vi "LaserLineDetection_Intensity_Gauss.vi"(6 "Color":u32(colorbox)=16744448, 8 "Error In":errorcluster, 10 "Point Information In":T1, 11 "Source In":T2=refnum) -> (0 "Error Out":errorcluster, 1 "appended array":cluster{u8[], i32[]}[](array[cluster]), 2 "Point Information Out":T1, 3 "Source Out":T2, 4 "Gauss Fit Accepted":bool, 5 "Intensity Average":u8)   [LabVIEW 2013]
uses:
  <vilib>/vision/Image Controls.llb/IMAQ Image.ctl
  Point Information.ctl
  <vilib>/Analysis/6fits.llb/Curve Fitting Criteria.ctl
  <vilib>/vision/NI_Vision_Development_Module.lvlib
  <vilib>/Analysis/NI_AALPro.lvlib
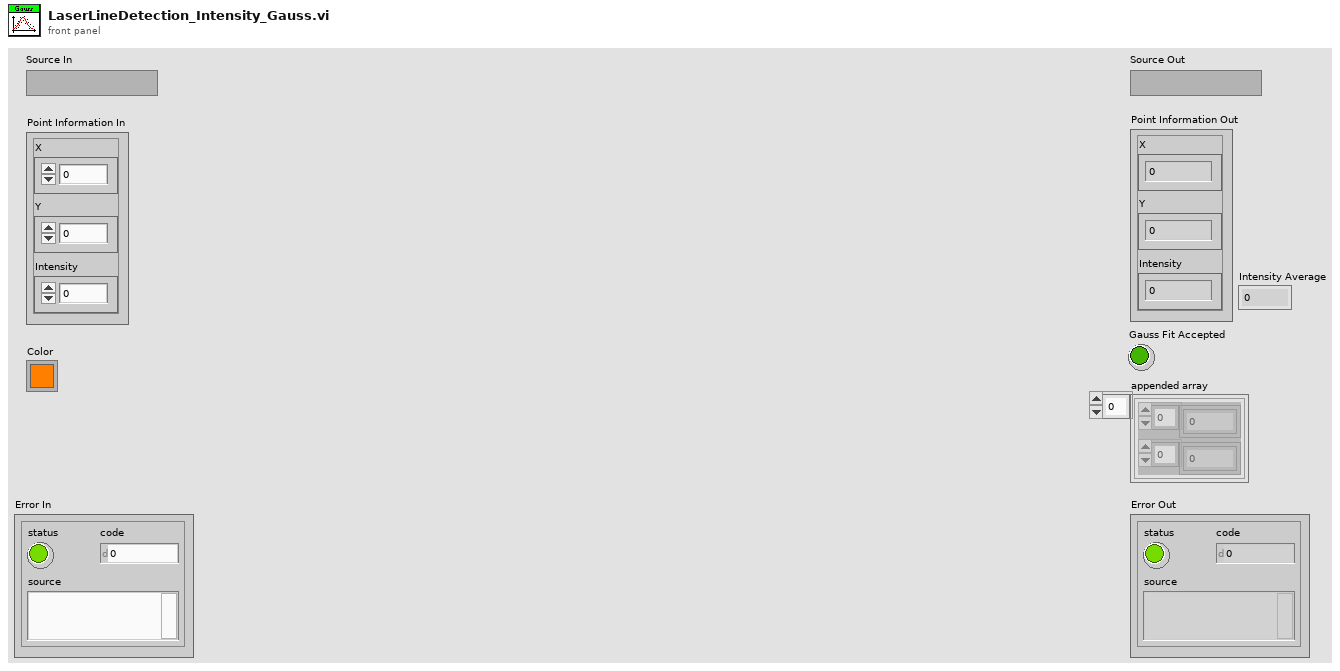
[diagram p1: front panel]
types:
  T1 = typedef "Point Information.ctl" = cluster{"X":i32, "Y":i32, "Intensity":u8}
  T2 = typedef "IMAQ Image.ctl" = refnum<image>
  T3 = cluster{"amp min":dbl, "amp max":dbl, "center min":dbl, "center max":dbl, "deviation min":dbl, "deviation max":dbl, "offset min":dbl, "offset max":dbl}
  T4 = typedef "NI_AALPro.lvlib/Curve Fitting Criteria.ctl" = u16
  T5 = cluster{"initial amplitude":dbl, "initial center":dbl, "initial standard deviation":dbl, "offset":dbl}
  T6 = cluster{"Red (or Hue) value":u8, "Green (or Sat) value":u8, "Blue (or Light or Val) value":u8}[]
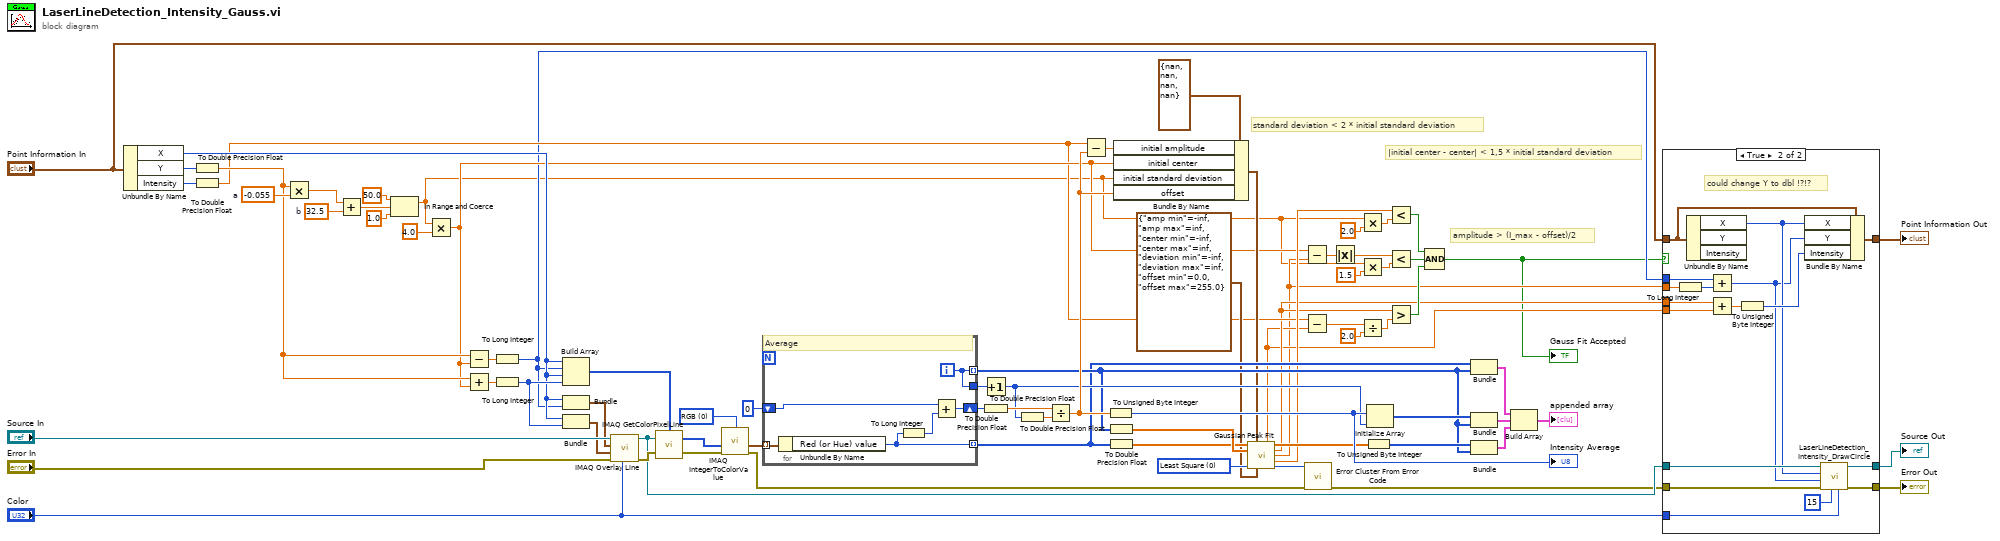
[diagram p0: block diagram]
diagram:
  w36 = T4 0 items=["Least Square", "Least Absolute Residual", "Bisquare"] ("method")
  w59 = 32.5  # b
  w61 = -0.055  # a
  w78 = u16 0 items=["RGB", "HSL", "HSV", "HSI"] ("Color Mode")
  # "amplitude > (I_max - offset)/2"
  # "|initial center - center| < 1,5 * initial standard deviation"
  # "standard deviation < 2 * initial standard deviation"
  n1 = Unbundle By Name("Point Information In") -> ("X"=w51:i32, "Y"=w50:i32, "Intensity"=w48:u8)
  n2 = To Double Precision Float(number=w50) -> (double precision float=w49:dbl)
  n3 = To Double Precision Float(number=w48) -> (double precision float=w23:dbl)
  n4 = Multiply(x=w49, y=w61) -> (x*y=w60:dbl)
  n5 = Add(x=w60, y=w59) -> (x+y=w8:dbl)
  n6 = In Range and Coerce(upper limit=50.0, x=w8, lower limit=1.0) -> (coerced(x)=w2:dbl)  [unwired: 1 out]
  n7 = Multiply(x=w2, y=4.0) -> (x*y=w27:dbl)
  n8 = Subtract(x=w49, y=w27) -> (x-y=w10:dbl)
  n9 = Add(x=w49, y=w27) -> (x+y=w57:dbl)
  n10 = To Long Integer(number=w10) -> (32bit integer=w9:i32)
  n11 = To Long Integer(number=w57) -> (32bit integer=w55:i32)
  n12 = Build Array(w51, w9, w51, w55) -> (w56:i32[])
  n13 = Bundle("X"=w51, w9) -> (w54:cluster{"X":i32, i32})  [unwired: 1 in]
  n14 = Bundle("X"=w51, w55) -> (w53:cluster{"X":i32, i32})  [unwired: 1 in]
  n15 = call "IMAQ Overlay Line"("Color"="Color", "error in (no error)"="Error In", "End Point"=w53, "Start Point"=w54, "Image"="Source In") -> ("error out"=w34:errorcluster, "Image Out"=w19:T2)  [unwired: 5 in]
  n16 = call "IMAQ GetColorPixelLine"("Line Coordinates"=w56, "Image"=w19, "error in (no error)"=w34) -> ("Pixels Line (U32)"=w77:u32[], "error out"=w33:errorcluster)  [unwired: 1 in, 1 out]
  n17 = call "IMAQ IntegerToColorValue"("error in (no error)"=w33, "1D U32 array"=w77, "Color Mode"=w78) -> ("1D Color value array"=w76:T6, "error out"=w64:errorcluster)  [unwired: 2 in, 2 out]
  n18 = for {
    tunnel: w76 -> [w84] mode=indexing
    shift-right: [w83] -> w45
    shift-left: 0 ("y") -> [w80]
    tunnel: [w82] -> w41 mode=indexing
    tunnel: [w81] -> w39 mode=indexing
    tunnel: [w82] -> w74
    i -> [w82]
    # "Average"
    n19 = Unbundle By Name(w84) -> ("Red (or Hue) value"=w81:u8)
    n20 = To Long Integer(number=w81) -> (32bit integer=w79:i32)
    n21 = Add(x=w80, y=w79) -> (x+y=w83:i32)
  }
  n22 = Increment(x=w74) -> (x+1=w43:i32)
  n23 = To Double Precision Float(number=w45) -> (double precision float=w44:dbl)
  n24 = To Double Precision Float(number=w43) -> (double precision float=w42:dbl)
  n25 = Divide(x=w44, y=w42) -> (x/y=w47:dbl)
  n26 = Subtract(x=w23, y=w47) -> (x-y=w46:dbl)
  n27 = To Unsigned Byte Integer(number=w47) -> (unsigned 8bit integer=w72:u8)
  "Intensity Average" <- w72
  n28 = To Double Precision Float(number=w41) -> (double precision float=w40:dbl[])
  n29 = To Double Precision Float(number=w39) -> (double precision float=w38:dbl[])
  n30 = Bundle By Name(cluster=T5 {"initial amplitude"=nan, "initial center"=nan, "initial standard deviation"=nan, "offset"=nan} ("initial guess"), "initial amplitude"=w46, "initial center"=w27, "initial standard deviation"=w2, "offset"=w47) -> (w37:T5)
  n31 = call <vilib>:"Gaussian Peak Fit.vi"("Y"=w38, "initial guess"=w37, "X"=w40, "method"=w36, "parameter bounds"=T3 {"amp min"=-inf, "amp max"=inf, "center min"=-inf, "center max"=inf, "deviation min"=-inf, "deviation max"=inf, "offset min"=0.0, "offset max"=255.0}) -> ("offset"=w12:dbl, "Best Gaussian Fit"=w70:dbl[], "amplitude"=w13:dbl, "center"=w11:dbl, "standard deviation"=w32:dbl, "error"=w68:i32)  [unwired: 4 in, 1 out]
  n32 = Subtract(x=w27, y=w11) -> (x-y=w29:dbl)
  n33 = Subtract(x=w23, y=w12) -> (x-y=w24:dbl)
  n34 = call <vilib>:"Error Cluster From Error Code.vi"("error in (no error)"=w64, "error code (0)"=w68) -> ("error out"=w18:errorcluster)  [unwired: 7 in]
  n35 = Absolute Value(x=w29) -> (abs(x)=w28:dbl)
  n36 = Multiply(x=w2, y=2.0) -> (x*y=w30:dbl)
  n37 = Multiply(x=w2, y=1.5) -> (x*y=w1:dbl)
  n38 = Divide(x=w24, y=2.0) -> (x/y=w26:dbl)
  n39 = To Unsigned Byte Integer(number=w70) -> (unsigned 8bit integer=w71:u8[])
  n40 = Initialize Array(w72, w43) -> (w69:u8[])
  n41 = Less?(x=w32, y=w30) -> (x < y?=w22:bool)
  n42 = Less?(x=w28, y=w1) -> (x < y?=w21:bool)
  n43 = Greater?(x=w13, y=w26) -> (0:w20:bool)
  n44 = Compound Arithmetic op=AND(w22, w21, w20) -> (w4:bool)
  "Gauss Fit Accepted" <- w4
  n45 = Bundle(w39, w41) -> (w67:cluster{u8[], i32[]})  [unwired: 1 in]
  n46 = Bundle(w69, w41) -> (w66:cluster{u8[], i32[]})  [unwired: 1 in]
  n47 = Bundle(w71, w41) -> (w65:cluster{u8[], i32[]})  [unwired: 1 in]
  n48 = Build Array(w67, w66, w65) -> (→"appended array":cluster{u8[], i32[]}[])
  n49 = case shown="True" w4 {
    tunnel: w18 -> [w86 w103]
    tunnel: w19 -> [w87 w102]
    tunnel: [w87 w101] -> w16
    tunnel: [w86 w100] -> w17
    tunnel: "Point Information In" -> [w85 w99]
    tunnel: [w85 w98] -> w14
    tunnel: w13 -> [_ w97]
    tunnel: w12 -> [_ w94]
    tunnel: w11 -> [_ w91]
    tunnel: w9 -> [_ w93]
    tunnel: "Color" -> [_ w88]
    frame False {
    }
    frame True {
      # "could change Y to dbl !?!?"
      n50 = To Long Integer(number=w91) -> (32bit integer=w92:i32)
      n51 = Unbundle By Name(w99) -> ("X"=w90:i32)  [unwired: 2 out]
      n52 = Add(x=w93, y=w92) -> (x+y=w89:i32)
      n53 = Add(x=w97, y=w94) -> (x+y=w96:dbl)
      n54 = To Unsigned Byte Integer(number=w96) -> (unsigned 8bit integer=w95:u8)
      n55 = Bundle By Name(cluster=w99, "X"=w90, "Y"=w89, "Intensity"=w95) -> (w98:T1)
      n56 = call "LaserLineDetection_Intensity_DrawCircle.vi"("Color"=w88, "Radius"=15, "Error In"=w103, "Y_center"=w89, "X_center"=w90, "Image in"=w102) -> ("Error Out"=w100:errorcluster, "Image out"=w101:T2)  [unwired: 4 in]
    }
  }
  "Source Out" <- w16
  "Error Out" <- w17
  "Point Information Out" <- w14
